vi "boxoverlayimage.vi"(3 "Image":T1, 4 "error in (no error)":errorcluster, 5 "ROI":i32=128, 6 "Array":i32[][](array[numeric])) -> (0 "error out":errorcluster, 2 "Image Out":T1)   [LabVIEW 2011]
uses:
  <vilib>/vision/Image Controls.llb/IMAQ Image.ctl
  <vilib>/vision/NI_Vision_Development_Module.lvlib
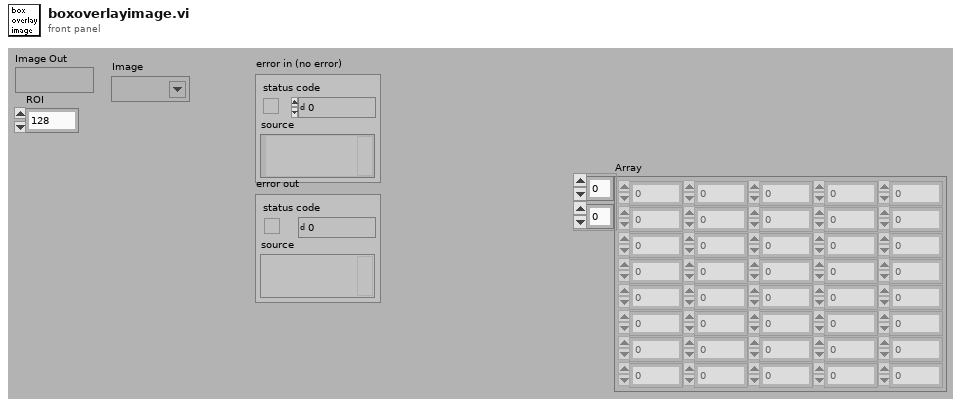
[diagram p1: front panel]
types:
  T1 = typedef "IMAQ Image.ctl" = refnum<image>
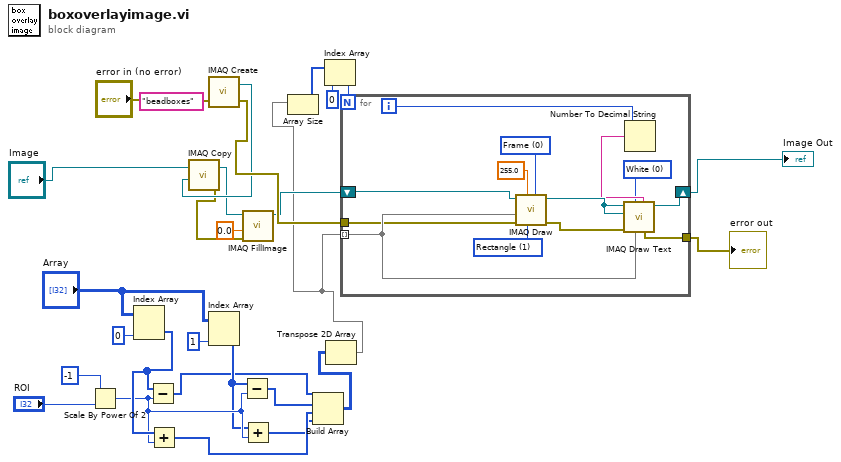
[diagram p0: block diagram]
diagram:
  n1 = Scale By Power Of 2(n=i16 -1, x="ROI") -> (x*2^n=w9:i32)
  n2 = Index Array(array="Array", index (col)=0 ("disabled index (col)")) -> (element=w10:i32[])  [unwired: 1 in]
  n3 = Subtract(x=w10, y=w9) -> (x-y=w7:i32[])
  n4 = Add(x=w10, y=w9) -> (x+y=w5:i32[])
  n5 = call "IMAQ Create"("Image Name"="beadboxes", "error in (no error)"="error in (no error)") -> ("New Image"=w21:T1, "error out"=w22:errorcluster)  [unwired: 2 in, 1 out]
  n6 = call "IMAQ Copy"("Image Dst"=w21, "Image Src"="Image") -> ("error out"=w20:errorcluster, "Image Dst Out"=w19:T1)  [unwired: 1 in, 3 out]
  n7 = Index Array(array="Array", index (col)=1 ("disabled index (col)")) -> (element=w8:i32[])  [unwired: 1 in]
  n8 = Subtract(x=w8, y=w9) -> (x-y=w6:i32[])
  n9 = call "IMAQ FillImage"("error in (no error)"=w20, "Pixel Value (U8, U16, I16, Float)"=sgl 0.0, "Image"=w19) -> ("Image Out"=w18:T1)  [unwired: 4 in, 4 out]
  n10 = Add(x=w8, y=w9) -> (x+y=w4:i32[])
  n11 = Build Array(w7, w6, w5, w4) -> (w2:i32[][])
  n12 = Transpose 2D Array(2D array=w2) -> (transposed array=w1:i32[][])
  n13 = Array Size(array=w1) -> (size(s)=w28:i32[])
  n14 = Index Array(array=w28, index=0) -> (element=w27:i32)
  n15 = for {
    N: w27 -> [_]
    tunnel: w1 -> [w37] mode=indexing
    shift-right: [w33] -> w15
    shift-left: w18 -> [w35]
    tunnel: [w34] -> w25
    tunnel: w22 -> [w32]
    i -> [w40]
    w30 = u16 0 items=["Frame", "Paint", "Invert Frame", "Invert Paint"] ("Draw Mode")
    w31 = u16 1 items=["Line", "Rectangle", "Oval"] ("Shape to draw")
    w38 = 0 items=["White", "Black", "Inverted", "Black on White", "White on Black"] ("Color")
    n16 = call "IMAQ Draw"("Draw Mode"=w30, "Shape to draw"=w31, "Pixel Color"=sgl 255.0, "error in (no error)"=w32, "Coordinates"=w37, "Image Src"=w35) -> ("error out"=w36:errorcluster, "Image Dst Out"=w41:T1)  [unwired: 1 in, 3 out]
    n17 = Number To Decimal String(number=w40) -> (decimal integer string=w39:string)  [unwired: 1 out]
    n18 = call "IMAQ Draw Text"("String"=w39, "Insertion Point"=w37, "Color"=w38, "error in (no error)"=w36, "Image Dst"=w41, "Image Src"=w41) -> ("error out"=w34:errorcluster, "Image Dst Out"=w33:T1)  [unwired: 1 in, 3 out]
  }
  "error out" <- w25
  "Image Out" <- w15
